vi "Do.vi"(8 "error in (no error)":errorcluster, 10 "Actor in":refnum<class "Actor.lvclass">, 11 "Update Time Msg":refnum<class "Update Time Event Msg.lvclass">) -> (0 "error out":errorcluster, 2 "Actor out":refnum<class "Actor.lvclass">)   [LabVIEW 2023, in "Example MVC Actors.lvlib" / "Example View.lvlib" / "Update Time Event Msg.lvclass"]
doc: "This VI delivers the message to the actor by calling the appropriate method(s) on the actor."
uses:
  Update Time Event Msg.lvclass
  C:/Projects/Shared Libraries/Event Actors/Event Handlers/Abstract Event Message for View/Abstract Event Message for View.lvclass
  <vilib>/ActorFramework/Actor/Actor.lvclass
  Example View/Example View.lvclass
  C:/Program Files/National Instruments/LabVIEW 2023/vi.lib/ActorFramework/Actor/Actor.lvclass
  Example Events/Timestamp Event.lvclass
  Event Handlers/Abstract Event Message for View/Abstract Event Message for View.lvclass/Abstract Event Message for View.ctl
  Example Events/Timestamp Event.lvclass/Timestamp Event.ctl
  Event Handlers/Abstract Event Message for View/Abstract Event Message for View.lvclass
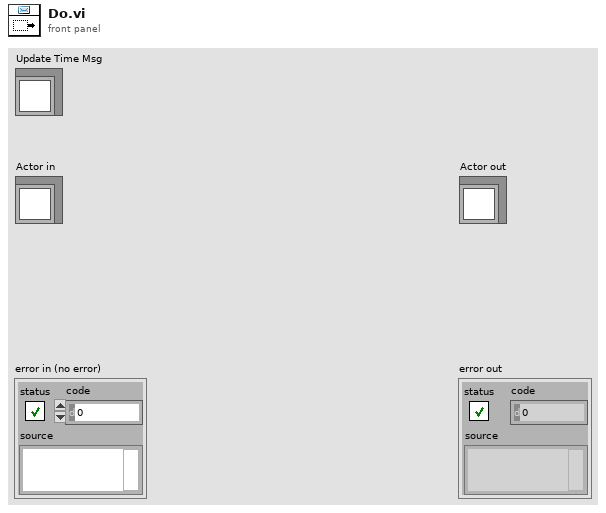
[diagram p1: front panel]
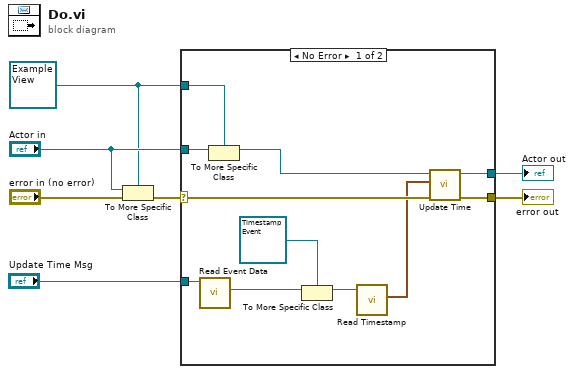
[diagram p0: block diagram]
diagram:
  w2 = refnum<class "Example View.lvclass"> refnum ("Actor in")
  n1 = To More Specific Class(target class=w2, reference="Actor in", error in="error in (no error)") -> (error out=w6:errorcluster)  [unwired: 1 out]
  n2 = case shown="No Error" w6 {
    selector: w6 -> [w16 w20]
    tunnel: [w18 w20] -> w5
    tunnel: [w17 w19] -> w4
    tunnel: "Actor in" -> [w15 w19]
    tunnel: w2 -> [w14 _]
    tunnel: "Update Time Msg" -> [w9 _]
    frame No Error {
      n3 = call "Read Event Data.vi"("Event Generated Msg"=w9) -> ("Event Data"=w8:refnum<class "Event.lvclass">)  [unwired: 10 in]
      n4 = To More Specific Class(target class=w14, reference=w15) -> (specific class reference=w13:refnum<class "Example View.lvclass">)  [unwired: 1 in, 1 out]
      n5 = To More Specific Class(target class=refnum<class "Timestamp Event.lvclass"> refnum ("Example Source.lvlib:Timestamp Event.lvclass"), reference=w8) -> (specific class reference=w11:refnum<class "Timestamp Event.lvclass">)  [unwired: 1 in, 1 out]
      n6 = call "Read Timestamp.vi"("Timestamp Event in"=w11) -> ("Timestamp"=w10:timestamp)  [unwired: 9 in, 1 out]
      n7 = call "Update Time.vi"("error in (no error)"=w16, "Timestamp"=w10, "Example View In"=w13) -> ("error out"=w18:errorcluster, "Example View Out"=w17:refnum<class "Example View.lvclass">)  [unwired: 7 in]
    }
    frame Error {
      # "If type check fails, pass the original object out again."
    }
  }
  "error out" <- w5
  "Actor out" <- w4
